vi "close_camera.vi"(0 "error":errorcluster, 8 "error 2":errorcluster, 11 "Handle":i32) -> ()   [LabVIEW 2019]
panel:
  in  "Apply Settings":bool
  in  "Centre AOI":bool
  in  "AOI Width":i64
  in  "AOI Height":i64
  out "Ready":bool
  in  "Run":bool
  out "Pixel Encoding":string
  out "AOIStride":i64
  in  "PreAmp Gain Control":string(combo)
  out "PixelData":u16[](array[numeric])
  out "ByteData":u8[](array[numeric])
  in  "ExposureTime":dbl=0.1
  out "ImageSizeBytes":i64
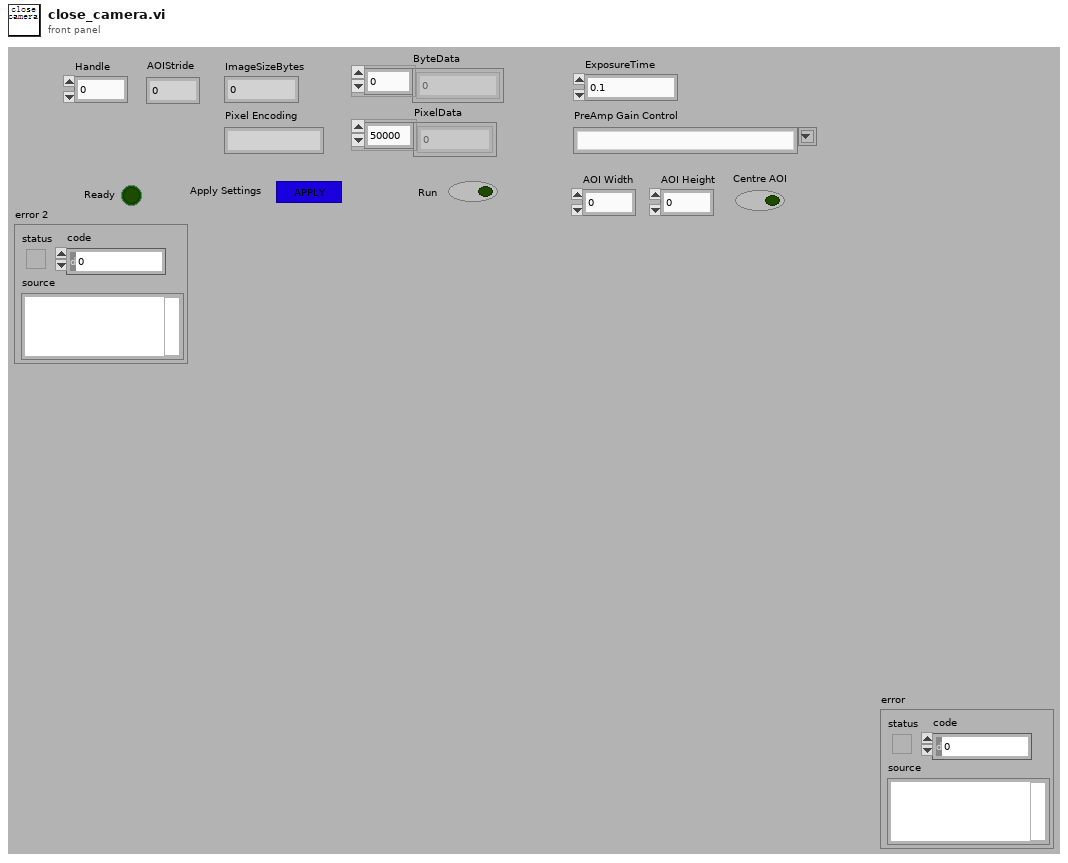
[diagram p1: front panel]
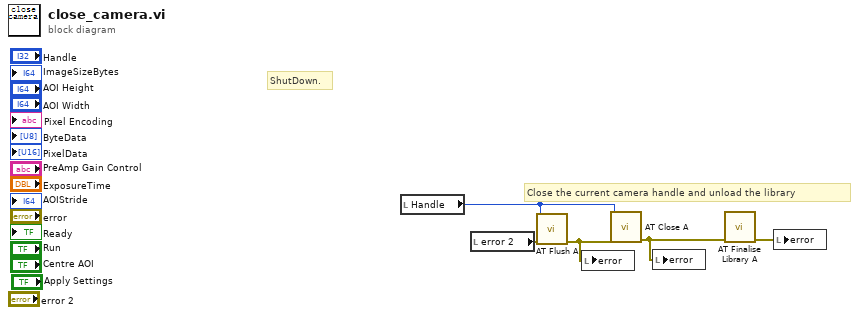
[diagram p0: block diagram]
diagram:
  # "Close the current camera handle and unload the library"
  # "ShutDown."
  n1 = local read "Handle"() -> (w1:i32)
  n2 = local read "error 2"() -> (w3:errorcluster)
  n3 = call <userlib>:"AT Flush A.vi"("error in (no error)"=w3, "Handle"=w1) -> ("error out"=w4:errorcluster)  [unwired: 8 in, 1 out]
  n4 = local write "error"(w4) -> ()
  n5 = call <userlib>:"AT Close A.vi"("error in (no error)"=w4, "Handle"=w1) -> ("error out"=w5:errorcluster)  [unwired: 8 in, 1 out]
  n6 = local write "error"(w5) -> ()
  n7 = call <userlib>:"AT Finalise Library A.vi"("error in (no error)"=w5) -> ("error out"=w2:errorcluster)  [unwired: 9 in, 1 out]
  n8 = local write "error"(w2) -> ()
